vi "LVClass_WavefrontCorrectorSet Save UsersParametersValue.vi"(0 "WavefrontCorrectorSet in":refnum<class "WavefrontCorrectorSet.lvclass">, 5 "ParametersValue file path":path, 11 "error in (no error)":errorcluster) -> (4 "WavefrontCorrectorSet out":refnum<class "WavefrontCorrectorSet.lvclass">, 15 "error out":errorcluster)   [LabVIEW 2020, in "WavefrontCorrectorSet.lvclass"]
uses:
  WavefrontCorrectorSet.lvclass
  WavefrontCorrectorSet.lvclass/WavefrontCorrectorSet.ctl
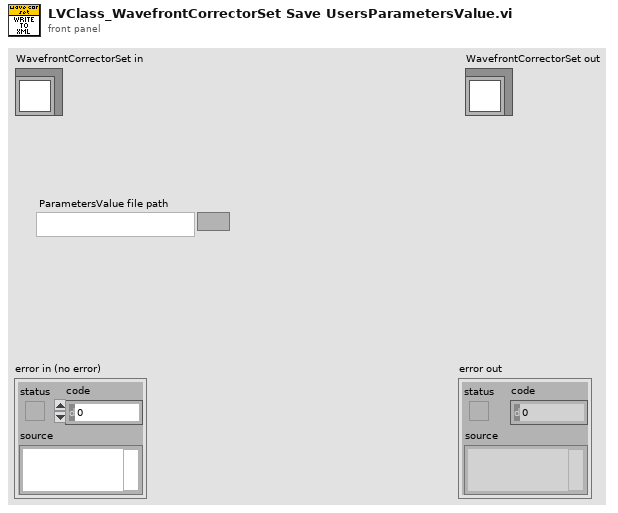
[diagram p1: front panel]
types:
  T1 = typedef "ClassID.ctl" = i64
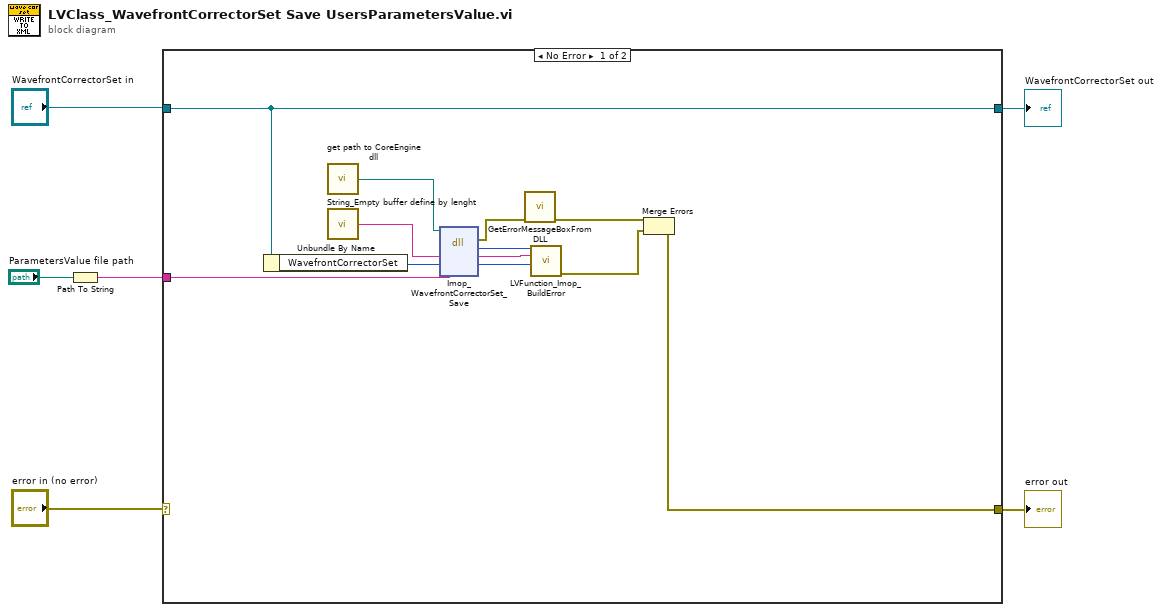
[diagram p0: block diagram]
diagram:
  n1 = Path To String(path="ParametersValue file path") -> (string=w1:string)
  n2 = case shown="No Error" "error in (no error)" {
    selector: "error in (no error)" -> [_ w20]
    tunnel: [w8 w20] -> w5
    tunnel: [w10 w19] -> w3
    tunnel: "WavefrontCorrectorSet in" -> [w10 w19]
    tunnel: w1 -> [w9 _]
    frame No Error {
      n3 = Unbundle By Name(w10) -> ("WavefrontCorrectorSet"=w18:T1)
      n4 = call "get path to CoreEngine dll.vi"() -> ("path to wavekit library"=w14:path)  [unwired: 14 in, 1 out]
      n5 = call "String_Empty buffer define by lenght.vi"() -> ("Empty buffer"=w11:string)  [unwired: 1 in]
      n6 = dll-call lib="D:/soft/HASO_v3/SVN_trunk/ImOpCoreEngine4_LV2011/DLLs/c_interface_vc100.dll" fn="Imop_WavefrontCorrectorSet_Save"(path in=w14, "message"=w11, "objet"=w18, "chemin_config"=w9) -> (error out=w15:errorcluster, "return type"=w13:i32, "message"=w12:string, "objet"=w7:i64)  [unwired: 3 in, 1 out]
      n7 = call "GetErrorMessageBoxFromDLL.vi"("error IN"=w15) -> ("error OUT"=w16:errorcluster)  [unwired: 10 in]
      n8 = call "LVFunction_Imop_BuildError.vi"("code"=w13, "String to Prepend to source (\"\")"=w12, "Adresse"=w7) -> ("error out"=w17:errorcluster)  [unwired: 12 in]
      n9 = Merge Errors(w16, w17) -> (w8:errorcluster)
    }
    frame Error {
    }
  }
  "error out" <- w5
  "WavefrontCorrectorSet out" <- w3
